vi "Read Channels and optional channel names.vi"(11 "Oscilloscope in":refnum<class "Oscilloscope.lvclass">) -> (2 "Channels and optional channel names":cluster{"Enabled":bool, "Channel name":string}[](array[cluster])=[{"Enabled"=TRUE, "Channel name"=""}, {"Enabled"=FALSE, "Channel name"=""}, {"Enabled"=FALSE, "Channel name"=""}, {"Enabled"=FALSE, "Channel name"=""}], 3 "Oscilloscope out":refnum<class "Oscilloscope.lvclass">)   [LabVIEW 2020, in "Oscilloscope.lvclass"]
uses:
  Oscilloscope.lvclass
  Oscilloscope.lvclass/Oscilloscope.ctl
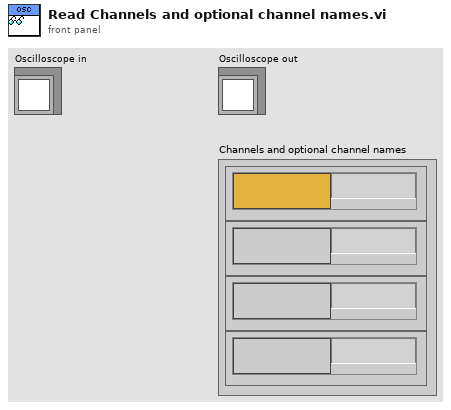
[diagram p1: front panel]
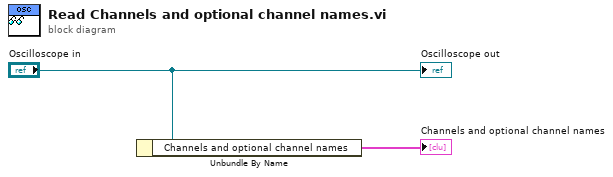
[diagram p0: block diagram]
diagram:
  n1 = Unbundle By Name("Oscilloscope in") -> ("Channels and optional channel names"=→"Channels and optional channel names":cluster{"Enabled":bool, "Channel name":string}[])
  "Oscilloscope out" <- "Oscilloscope in"
